vi "BioFeedback13(Small Buckets + Envelope).vi"(7 "Frames Per Second":dbl=30.0, 9 "Start Trial":bool, 11 "End Trial":bool, 12 "Data Directory":path, 13 "File Name":string, 14 "Extension":string="_EMG.txt") -> ()   [LabVIEW 2016]
uses:
  <vilib>/Utility/error.llb/DialogType.ctl
  <vilib>/Waveform/WDTOps.llb/WDT Append Waveforms DBL.vi
  <vilib>/Waveform/WDTFileIO.llb/Export Waveforms To Spreadsheet File (1D).vi
  <vilib>/Utility/file.llb/Write Delimited Spreadsheet (string).vi
panel:
  out "EndProcessTic":u32
  out "StartProcessTic":u32
  out "EndRecordTic":u32
  out "startRecordTic":u32
  out "Start UI":timestamp
  out "UI Elapsed Time":u32
  out "End UI":timestamp
  out "End Process":timestamp
  out "Start Process":timestamp
  out "End Record":timestamp
  out "Start Record":timestamp
  out "Process Elapsed Time":u32
  out "Record Elapsed Time":u32
  out "FilteredTrialData":waveform(dbl)[](graph)
  out "FilteredAndRectified":waveform(dbl)[](graph) caption="Filtered and Rectified"
  out "FilteredTrialData":waveform(dbl)[](array[waveform])
  in  "DisplayChannel":dbl
  out "BigWindowTrialData":dbl[][](array[numeric])
  out "DisplayValueByChannel":dbl[](array[numeric])
  out "RmsBufferSize":dbl
  out "RmsBufferIndices":dbl[](array[numeric])
  in  "Big Window Length (s)":dbl=0.5
  out "RmsBuffers":dbl[][](array[numeric])
  out "SmallWindowTrialData":dbl[][](array[numeric])
  out "CurrentRMSByChannel":dbl[](array[numeric])
  out "FilteredBuffer":dbl[][](array[numeric])
  out "Trial Data Column Headers":string[](array[string])
  in  "TrialDataRowHeaders":string[](array[string])=["Wfm1", "Wfm2", "Wfm3", "Wfm4", "Wfm5", "Wfm6", "Wfm7", "Wfm8"]
  out "GetMaxStartTime":timestamp
  in  "SecondsToAcquireMax":dbl=10.0
  in  "NumberOfMaximumsToTake":dbl=3.0
  in  "CurrentMaxIndex":dbl
  out "SignalsMaxArray":dbl[](array[numeric])
  out "SignalMaxTrialsArray":dbl[][](array[numeric])
  in  "%StdDevIndex":dbl=5.0
  in  "Mean%Index":dbl=4.0
  in  "StdDevIndex":dbl=3.0
  in  "MeanIndex":dbl=2.0
  in  "MaxIndex":dbl=1.0
  in  "MinIndex":dbl
  out "Stability Data":dbl[][](array[numeric])
  out "RawTrialData":waveform(dbl)[](array[waveform])
  in  "UI Ampl Error Path":path=path "C:/Users/Tinggroup/Desktop/VRMuscleActivationVisualizer/VRBiofeedback_v2/assets/BiofeedbackAmplitudeError.txt"
  out "DisplayActivation":dbl
  out "Acquiring Max":bool
  in  "resetMax":bool
  in  "startGetMax":bool
  in  "Amplitude Error":dbl
  in  "UI Data Path":path=path "C:/Users/Tinggroup/Desktop/VRMuscleActivationVisualizer/VRBiofeedback_v2/assets/LeftEMGData.txt"
  in  "EMG Input Device\nProduct Type":string="USB-6009"
  out "DisplayBarActivation":dbl(slide) caption="Left" max=1.0 scale=0.0..100.0
  out "Processed8":dbl[](graph)
  out "Processsed7":dbl[](graph)
  out "Processed6":dbl[](graph)
  out "Processed5":dbl[](graph)
  out "Processed4":dbl[](graph)
  out "Processed3":dbl[](graph)
  out "Processed2":dbl[](graph)
  out "Processed1":dbl[](graph)
  out "Raw Trial Data Wfm":waveform(dbl)[](graph)
  in  "UI Percent Path":path=path "C:/Users/Tinggroup/Desktop/VRMuscleActivationVisualizer/VRBiofeedback_v2/assets/BiofeedbackTargetPercentage.txt"
  in  "Target Percentage":dbl=10.0
  out "Trial In Progress":bool
  in  "Lower Cut-Off":dbl=20.0
  in  "Upper Cut-Off":dbl=300.0
  out "raw data":dynamicdata(graph)
  out "FilteredBufferIndices":dbl[](array[numeric])
  out "FilteredBufferSize":dbl
  out "Samples per frame":dbl
  out "Reset Data Acquisition\nAnd UI Updating":bool=TRUE
  in  "Small Window Length (s)":dbl=0.5
  in  "Sample rate (Hz)":dbl=2000.0
  in  "End Program":bool
  # "Saving Trial Data"
  # "Filter and Process Parameters"
  # "Set Target"
  # "Changes are made instantly and cause moving average to reset to zero"
  # "Scale Max"
  # "Channels used in Display"
  # "Analyze Stability of Displayed Data"
  # "Auto Analyze Stability begins calculating stability\nAs soon as dot enters the target zone and stops \nonce the dot leaves the target zone (Not Yet Implemented)"
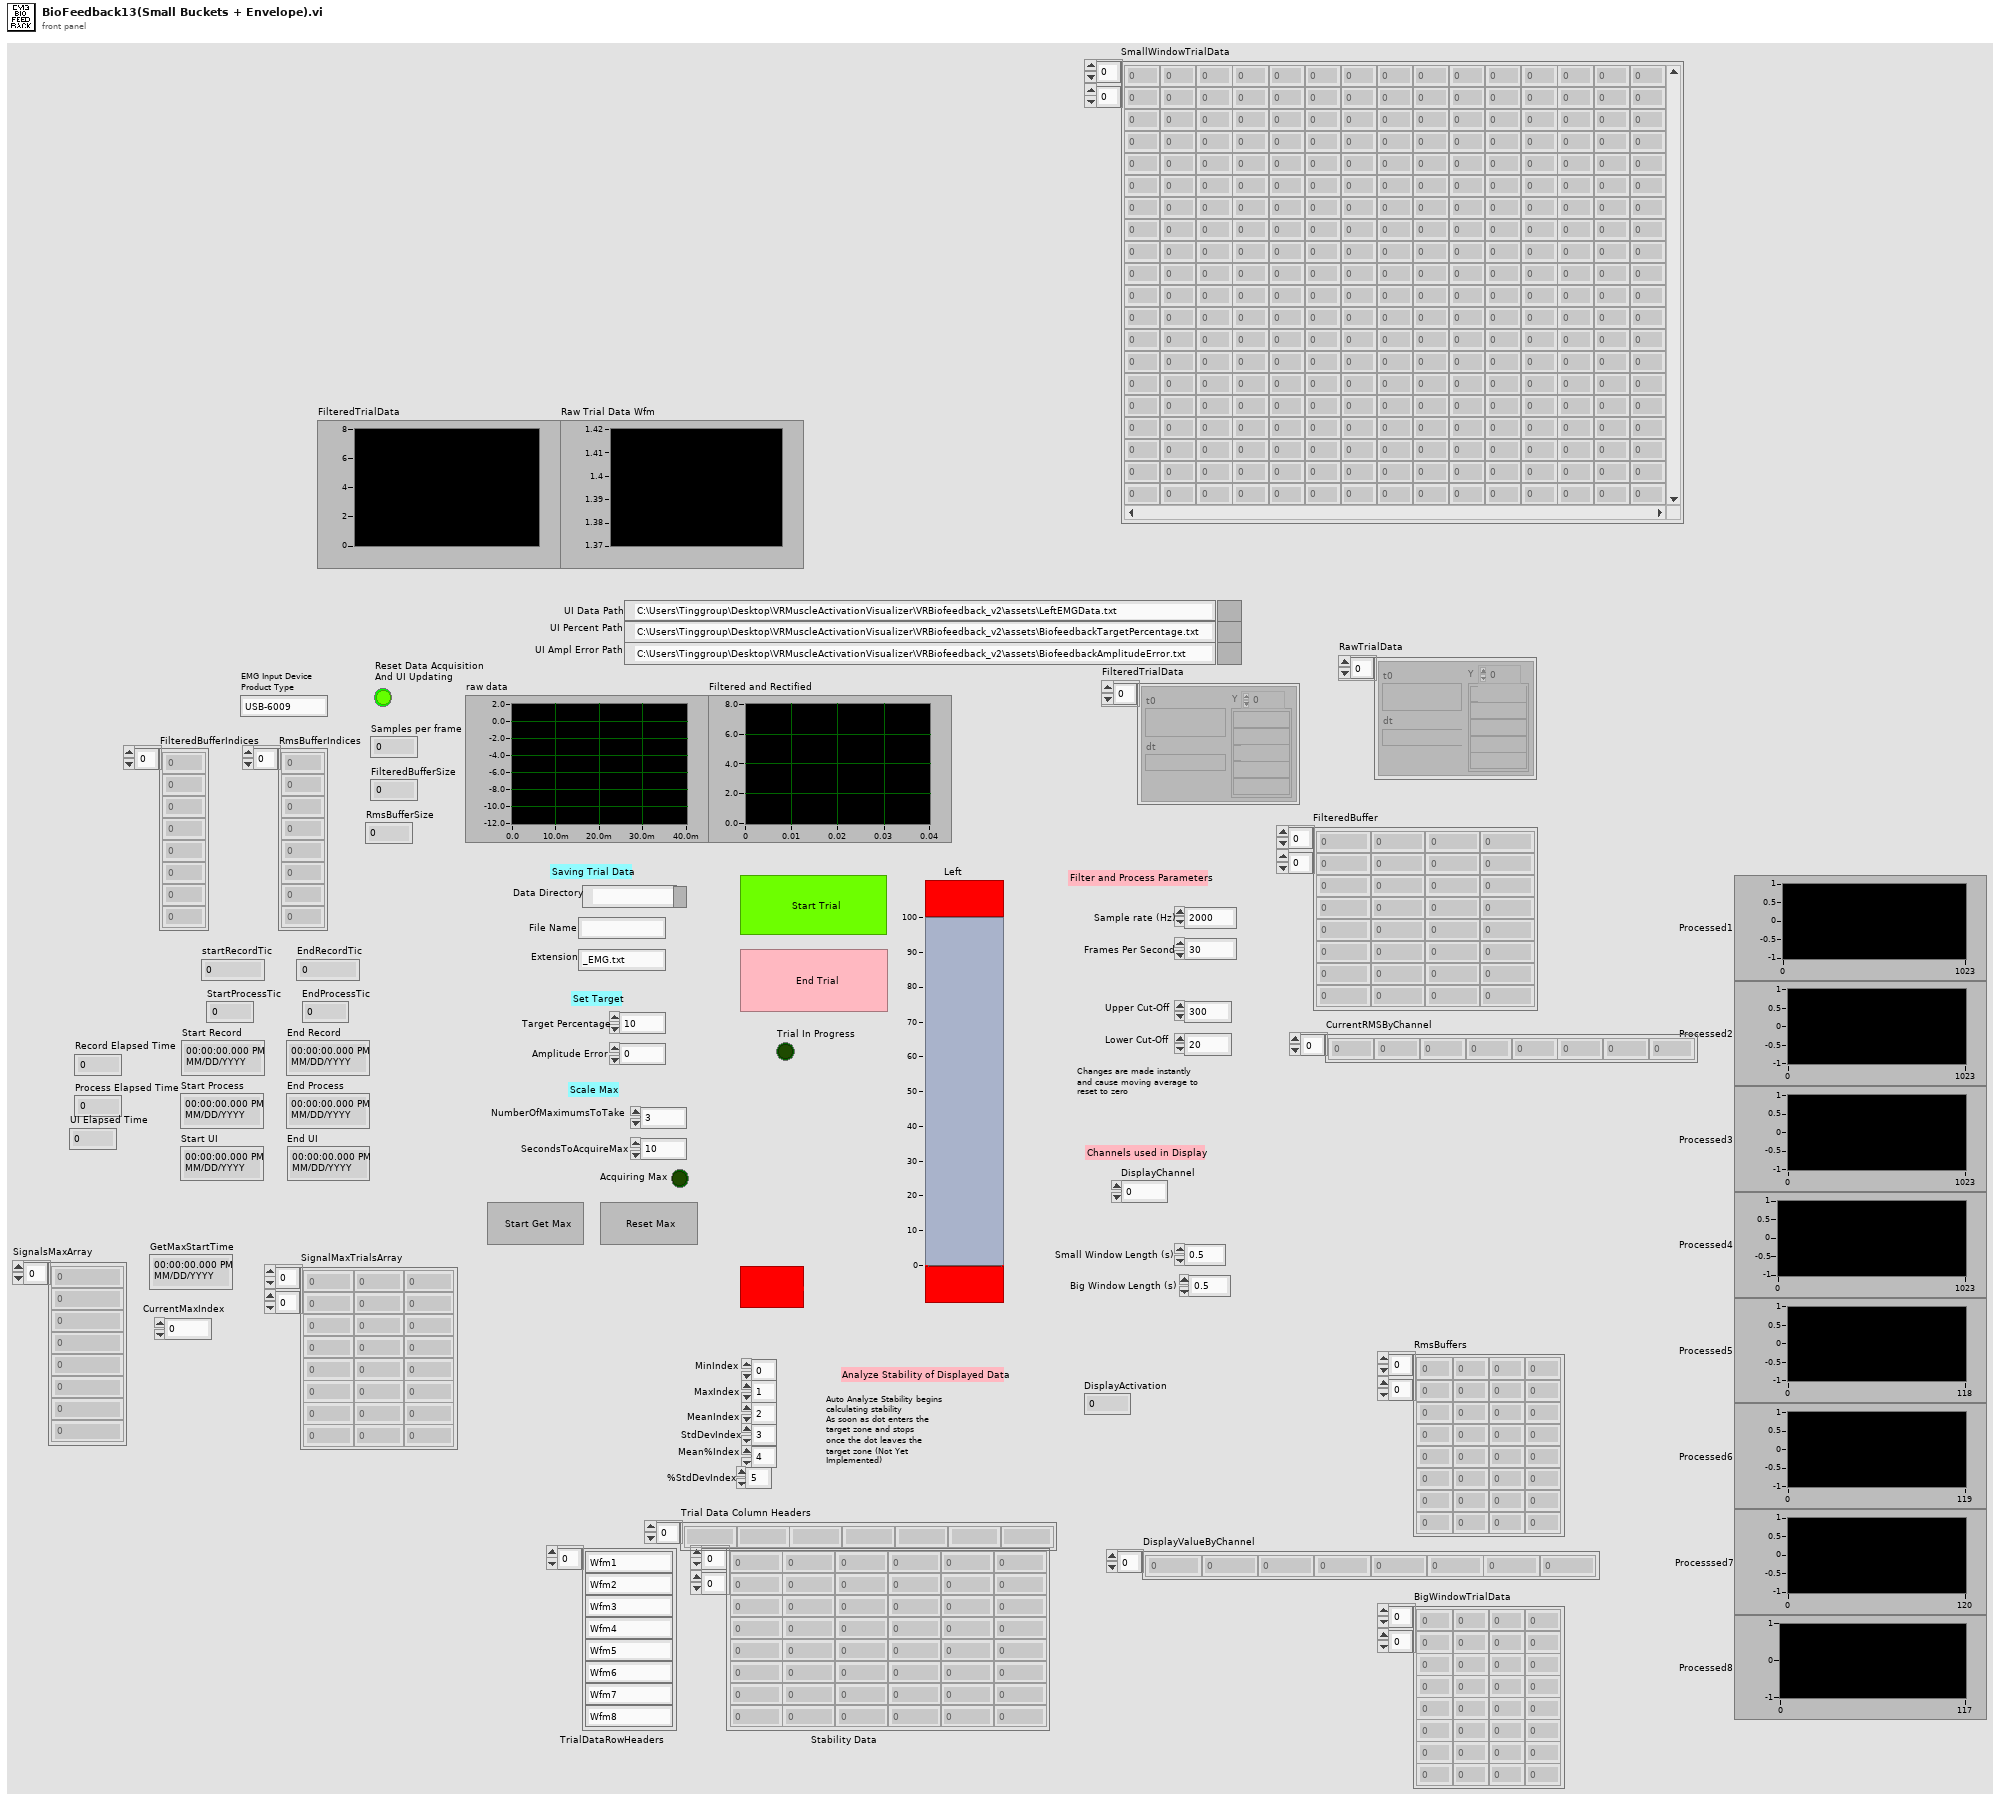
[diagram p1: front panel]
types:
  T1 = typedef "DialogType.ctl" = u16
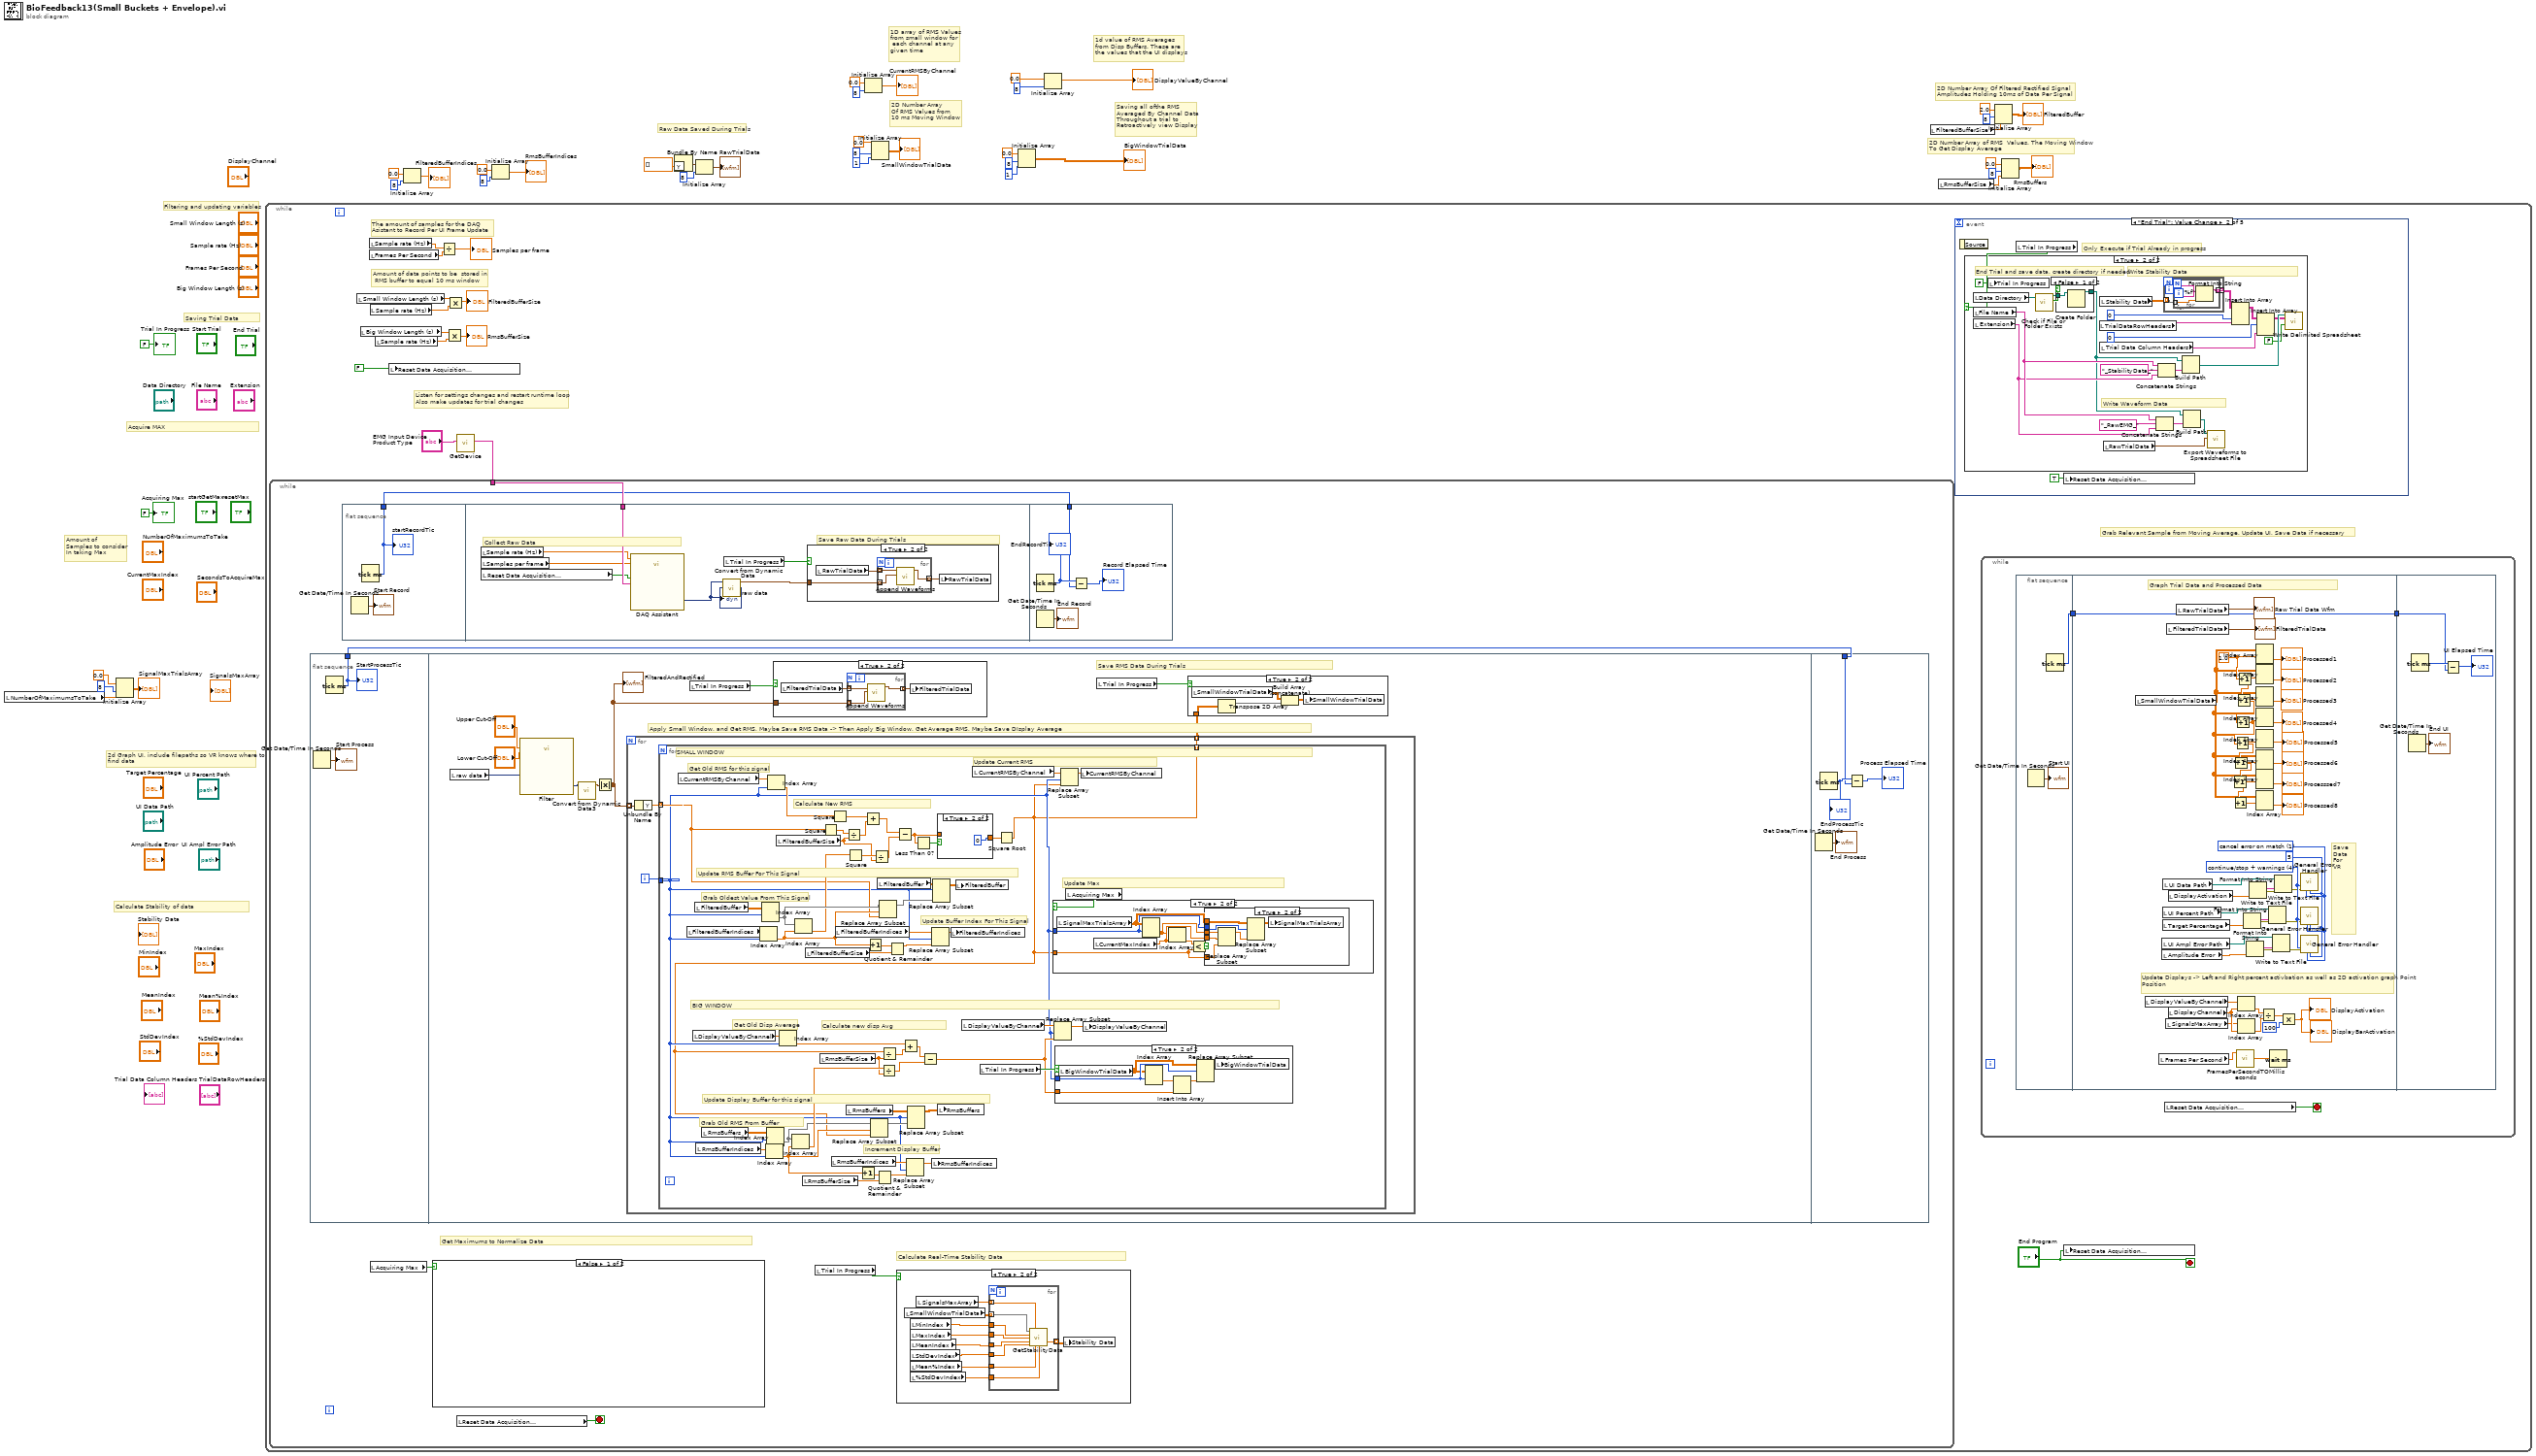
[diagram p0: block diagram]
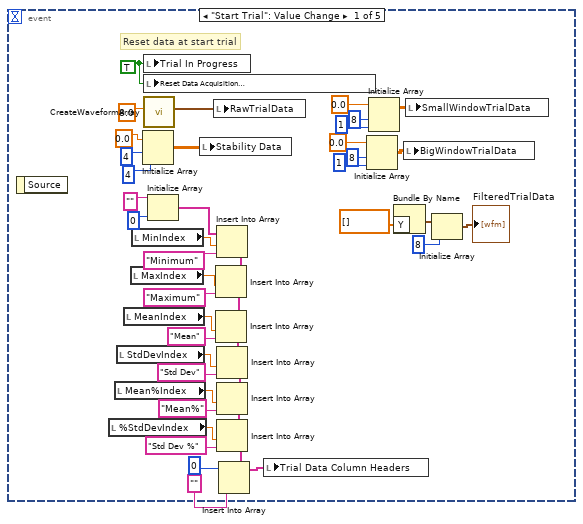
[diagram p2: hidden frame]
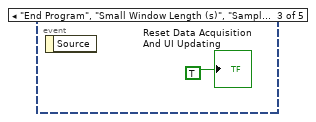
[diagram p5: hidden frame]
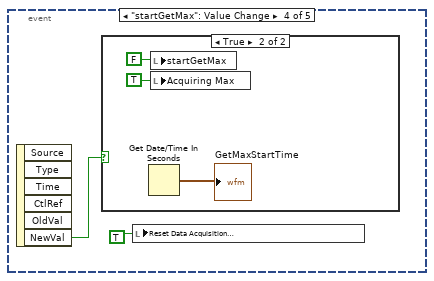
[diagram p6: hidden frame]
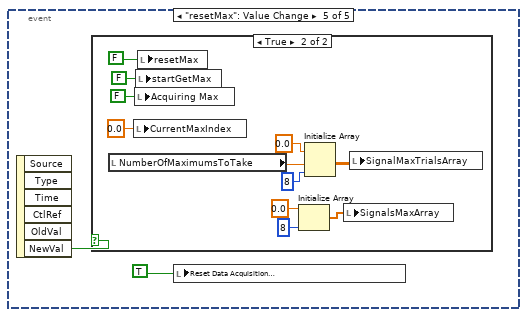
[diagram p8: hidden frame]
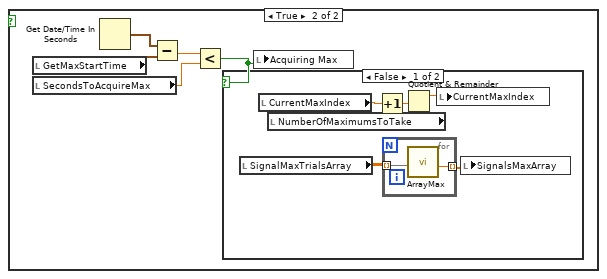
[diagram p17: hidden frame]
diagram:
  # "2D Number Array of RMS  Values. The Moving Window To Get Display Average"
  # "2D Number Array Of Filtered Rectified Signal Amplitudes Holding 10ms of Data Per Signal"
  # "Saving all ofthe RMS\nAveraged By Channel Data\nThroughout a trial to \nRetroactively view Display"
  # "1d value of RMS Averages\nfrom Disp Buffers. These are\nthe values that the UI displays"
  # "1D array of RMS Values\nfrom small window for\n each channel at any\ngiven time"
  # "2D Number Array\nOf RMS Values from\n10 ms Moving Window"
  # "Raw Data Saved During Trials"
  # "Amount of \nSamples to consider\nIn taking Max"
  # "Calculate Stability of data"
  # "Acquire MAX"
  # "Filtering and updating variables"
  # "Saving Trial Data"
  # "2d Graph UI, include filepaths so VR knows where to find data"
  n1 = local read "NumberOfMaximumsToTake"() -> (w12:dbl)
  n2 = Initialize Array(0.0 ("element"), 8 ("dimension size"), w12) -> (→"SignalMaxTrialsArray":dbl[][])
  n3 = while {
    stop <- "End Program" stop-if-true
    # "Grab Relevant Sample from Moving Average, Update UI, Save Data if necessary"
    # "Amount of data points to be  stored in\n RMS buffer to equal 10 ms window"
    # "The amount of samples for the DAQ Asistant to Record Per UI Frame Update"
    # "Listen for settings changes and restart runtime loop\nAlso make updates for trial changes"
    n4 = local read "Small Window Length (s)"() -> (w43:dbl)
    n5 = local read "Big Window Length (s)"() -> (w41:dbl)
    n6 = local read "Sample rate (Hz)"() -> (w51:dbl)
    n7 = local read "Frames Per Second"() -> (w50:dbl)
    n8 = local read "Sample rate (Hz)"() -> (w44:dbl)
    n9 = local read "Sample rate (Hz)"() -> (w40:dbl)
    n10 = local write "Reset Data Acquisition\nAnd UI Updating"(FALSE) -> ()
    n11 = Divide(x=w51, y=w50) -> (x/y=→"Samples per frame":dbl)
    n12 = Multiply(x=w41, y=w40) -> (x*y=→"RmsBufferSize":dbl)
    n13 = Multiply(x=w43, y=w44) -> (x*y=→"FilteredBufferSize":dbl)
    n14 = call "GetDevice.vi"("EMG Input Device\nProduct Type"="EMG Input Device\nProduct Type") -> ("DAQmx Device Name"=w45:tag)  [unwired: 10 in]
    n15 = while {
      tunnel: w45 -> [w209]
      stop <- w204 stop-if-true
      # "Calculate Real-Time Stability Data"
      # "Get Maximums to Normalize Data"
      n16 = flat-sequence {
        tunnel: [w211] -> w206
        tunnel: w206 -> [w312]
        frame #0 {
          n17 = Get Date/Time In Seconds() -> (seconds since 1Jan1904=→"Start Process":timestamp)
          n18 = Tick Count (ms)() -> (millisecond timer value=w211:u32)
          "StartProcessTic" <- w211
        }
        frame #1 {
          # "Save RMS Data During Trials"
          # "Apply Small Window, and Get RMS, Maybe Save RMS Data -> Then Apply Big Window, Get Average RMS, Maybe Save DIsplay Average"
          n19 = local read "raw data"() -> (w220:dynamicdata)
          n20 = call "Filter"("Lower Cut-Off"="Lower Cut-Off", "Upper Cut-Off"="Upper Cut-Off", "Signal"=w220) -> ("Filtered Signal"=w219:dynamicdata)  [unwired: 7 in, 1 out]
          n21 = call "Convert from Dynamic Data3"("Dynamic Data Type"=w219) -> ("Array of Waveform"=w218:waveform(dbl)[])  [unwired: 3 in]
          n22 = Absolute Value(x=w218) -> (abs(x)=w214:waveform(dbl)[])
          "FilteredAndRectified" <- w214
          n23 = for {
            tunnel: w214 -> [w228] mode=indexing
            tunnel: [w225] -> w212 mode=indexing
            i -> [w226]
            n24 = Unbundle By Name(w228) -> ("Y"=w227:dbl[])
            n25 = for {
              tunnel: w227 -> [w238] mode=indexing
              tunnel: w226 -> [w230]
              tunnel: [w229] -> w225 mode=indexing
              # "Update Max"
              # "SMALL WINDOW"
              # "BIG WINDOW"
              # "Increment Display Buffer"
              # "Get Old Disp Average"
              # "Calculate new disp Avg"
              # "Grab Old RMS From Buffer"
              # "Update Display Buffer for this signal"
              # "Update Buffer Index For This Signal"
              # "Update RMS Buffer For This Signal"
              # "Update Current RMS"
              # "Calculate New RMS"
              # "Grab Oldest Value From This Signal"
              # "Get Old RMS for this signal"
              n26 = local read "CurrentRMSByChannel"() -> (w261:dbl[])
              n27 = local read "FilteredBufferIndices"() -> (w266:dbl[])
              n28 = local read "DisplayValueByChannel"() -> (w255:dbl[])
              n29 = local read "FilteredBuffer"() -> (w262:dbl[][])
              n30 = local read "RmsBufferIndices"() -> (w249:dbl[])
              n31 = local read "RmsBuffers"() -> (w258:dbl[][])
              n32 = Index Array(array=w266, index=w230) -> (element=w256:dbl)
              n33 = Index Array(array=w262, index (row)=w230) -> (element=w270:dbl[])  [unwired: 1 in]
              n34 = Index Array(array=w249, index=w230) -> (element=w241:dbl)
              n35 = Index Array(array=w258, index (row)=w230) -> (element=w235:dbl[])  [unwired: 1 in]
              n36 = Index Array(array=w261, index=w230) -> (element=w275:dbl)
              n37 = local read "FilteredBufferSize"() -> (w280:dbl)
              n38 = Index Array(array=w255, index=w230) -> (element=w246:dbl)
              n39 = Index Array(array=w235, index=w241) -> (element=w248:dbl)
              n40 = Index Array(array=w270, index=w256) -> (element=w254:dbl)
              n41 = local read "RmsBufferSize"() -> (w260:dbl)
              n42 = local read "FilteredBufferSize"() -> (w268:dbl)
              n43 = local read "RmsBufferSize"() -> (w245:dbl)
              n44 = Square(x=w238) -> (x^2=w282:dbl)
              n45 = Square(x=w275) -> (x^2=w279:dbl)
              n46 = local read "RmsBufferIndices"() -> (w240:dbl[])
              n47 = local read "FilteredBufferIndices"() -> (w263:dbl[])
              n48 = Divide(x=w282, y=w280) -> (x/y=w278:dbl)
              n49 = local read "RmsBuffers"() -> (w251:dbl[][])
              n50 = Square(x=w254) -> (x^2=w281:dbl)
              n51 = Increment(x=w241) -> (x+1=w259:dbl)
              n52 = Add(x=w279, y=w278) -> (x+y=w277:dbl)
              n53 = Increment(x=w256) -> (x+1=w267:dbl)
              n54 = Divide(x=w281, y=w280) -> (x/y=w276:dbl)
              n55 = Quotient & Remainder(x=w259, y=w260) -> (x-y*floor(x/y)=w239:dbl)  [unwired: 1 out]
              n56 = local read "FilteredBuffer"() -> (w271:dbl[][])
              n57 = Replace Array Subset(array=w270, new element=w238, index=w256) -> (w274:dbl[])
              n58 = Divide(x=w248, y=w245) -> (x/y=w252:dbl)
              n59 = Quotient & Remainder(x=w267, y=w268) -> (x-y*floor(x/y)=w264:dbl)  [unwired: 1 out]
              n60 = Subtract(x=w277, y=w276) -> (x-y=w233:dbl)
              n61 = Replace Array Subset(array=w240, new element=w239, index=w230) -> (w237:dbl[])
              n62 = Less Than 0?(x=w233) -> (x < 0?=w234:bool)
              n63 = Replace Array Subset(array=w263, new element=w264, index=w230) -> (w265:dbl[])
              n64 = local write "RmsBufferIndices"(w237) -> ()
              n65 = Replace Array Subset(array=w271, new element=w274, index (row)=w230) -> (w269:dbl[][])  [unwired: 1 in]
              n66 = case shown="True" w234 {
                tunnel: w233 -> [w297 _]
                tunnel: [w297 0] -> w232
                frame False {
                }
                frame True {
                }
              }
              n67 = local write "FilteredBufferIndices"(w265) -> ()
              n68 = local write "FilteredBuffer"(w269) -> ()
              n69 = local read "DisplayValueByChannel"() -> (w244:dbl[])
              n70 = local read "CurrentRMSByChannel"() -> (w273:dbl[])
              n71 = local read "Trial In Progress"() -> (w242:bool)
              n72 = Square Root(x=w232) -> (sqrt(x)=w229:dbl)
              n73 = Replace Array Subset(array=w235, new element=w229, index=w241) -> (w250:dbl[])
              n74 = Divide(x=w229, y=w245) -> (x/y=w247:dbl)
              n75 = Add(x=w246, y=w247) -> (x+y=w253:dbl)
              n76 = Replace Array Subset(array=w251, new element=w250, index (row)=w230) -> (w257:dbl[][])  [unwired: 1 in]
              n77 = Subtract(x=w253, y=w252) -> (x-y=w236:dbl)
              n78 = local write "RmsBuffers"(w257) -> ()
              n79 = Replace Array Subset(array=w244, new element=w236, index=w230) -> (w243:dbl[])
              n80 = case shown="True" w242 {
                tunnel: w230 -> [_ w302]
                tunnel: w236 -> [_ w303]
                frame False {
                }
                frame True {
                  n81 = local read "BigWindowTrialData"() -> (w301:dbl[][])
                  n82 = Index Array(array=w301, index (row)=w302) -> (element=w304:dbl[])  [unwired: 1 in]
                  n83 = Insert Into Array(array=w304, new element=w303) -> (w300:dbl[])  [unwired: 1 in]
                  n84 = Replace Array Subset(array=w301, new element=w300, index (row)=w302) -> (w299:dbl[][])  [unwired: 1 in]
                  n85 = local write "BigWindowTrialData"(w299) -> ()
                }
              }
              n86 = Replace Array Subset(array=w273, new element=w229, index=w230) -> (w272:dbl[])
              n87 = local read "Acquiring Max"() -> (w231:bool)
              n88 = case shown="True" w231 {
                tunnel: w230 -> [_ w283]
                tunnel: w229 -> [_ w286]
                frame False {
                }
                frame True {
                  n89 = local read "SignalMaxTrialsArray"() -> (w284:dbl[][])
                  n90 = local read "CurrentMaxIndex"() -> (w287:dbl)
                  n91 = Index Array(array=w284, index (row)=w283) -> (element=w285:dbl[])  [unwired: 1 in]
                  n92 = Index Array(array=w285, index=w287) -> (element=w289:dbl)
                  n93 = Less?(x=w289, y=w286) -> (x < y?=w288:bool)
                  n94 = case shown="True" w288 {
                    tunnel: w287 -> [_ w296]
                    tunnel: w286 -> [_ w295]
                    tunnel: w285 -> [_ w294]
                    tunnel: w284 -> [_ w293]
                    tunnel: w283 -> [_ w292]
                    frame False {
                    }
                    frame True {
                      n95 = Replace Array Subset(array=w294, new element=w295, index=w296) -> (w291:dbl[])
                      n96 = Replace Array Subset(array=w293, new element=w291, index (row)=w292) -> (w290:dbl[][])  [unwired: 1 in]
                      n97 = local write "SignalMaxTrialsArray"(w290) -> ()
                    }
                  }
                }
              }
              n98 = local write "CurrentRMSByChannel"(w272) -> ()
              n99 = local write "DisplayValueByChannel"(w243) -> ()
            }
          }
          n100 = local read "Trial In Progress"() -> (w215:bool)
          n101 = case shown="True" w215 {
            tunnel: w214 -> [_ w306]
            frame False {
            }
            frame True {
              n102 = local read "FilteredTrialData"() -> (w307:waveform(dbl)[])
              n103 = for {
                tunnel: w307 -> [w310] mode=indexing
                tunnel: w306 -> [w309] mode=indexing
                tunnel: [w308] -> w305 mode=indexing
                n104 = call-poly <vilib>:"Append Waveforms.vi"("waveform B"=w309, "waveform A"=w310) -> ("waveform out"=w308:waveform(dbl))  [unwired: 8 in, 1 out]
              }
              n105 = local write "FilteredTrialData"(w305) -> ()
            }
          }
          n106 = local read "Trial In Progress"() -> (w213:bool)
          n107 = case shown="True" w213 {
            tunnel: w212 -> [_ w221]
            frame False {
            }
            frame True {
              n108 = local read "SmallWindowTrialData"() -> (w222:dbl[][])
              n109 = Transpose 2D Array(2D array=w221) -> (transposed array=w224:dbl[][])
              n110 = Build Array (concatenate)(w222, w224) -> (w223:dbl[][])
              n111 = local write "SmallWindowTrialData"(w223) -> ()
            }
          }
        }
        frame #2 {
          n112 = Get Date/Time In Seconds() -> (seconds since 1Jan1904=→"End Process":timestamp)
          n113 = Tick Count (ms)() -> (millisecond timer value=w313:u32)
          "EndProcessTic" <- w313
          n114 = Subtract(x=w313, y=w312) -> (x-y=→"Process Elapsed Time":u32)
        }
      }
      n115 = flat-sequence {
        tunnel: [w316] -> w205
        tunnel: w209 -> [w323]
        tunnel: w205 -> [w330]
        frame #0 {
          n116 = Get Date/Time In Seconds() -> (seconds since 1Jan1904=→"Start Record":timestamp)
          n117 = Tick Count (ms)() -> (millisecond timer value=w316:u32)
          "startRecordTic" <- w316
        }
        frame #1 {
          # "Save Raw Data During Trials"
          # "Collect Raw Data"
          n118 = local read "Sample rate (Hz)"() -> (w319:dbl)
          n119 = local read "Samples per frame"() -> (w318:dbl)
          n120 = local read "Reset Data Acquisition\nAnd UI Updating"() -> (w317:bool)
          n121 = call "DAQ Assistant"("rate"=w319, "number of samples"=w318, "stop (T)"=w317, "device name"=w323) -> ("data"=w321:dynamicdata)  [unwired: 13 in, 2 out]
          "raw data" <- w321
          n122 = call "Convert from Dynamic Data"("Dynamic Data Type"=w321) -> ("Array of Waveform"=w320:waveform(dbl)[])  [unwired: 3 in]
          n123 = local read "Trial In Progress"() -> (w322:bool)
          n124 = case shown="True" w322 {
            tunnel: w320 -> [_ w326]
            frame False {
            }
            frame True {
              n125 = local read "RawTrialData"() -> (w325:waveform(dbl)[])
              n126 = for {
                tunnel: w326 -> [w328] mode=indexing
                tunnel: w325 -> [w329] mode=indexing
                tunnel: [w327] -> w324 mode=indexing
                n127 = call-poly <vilib>:"Append Waveforms.vi"("waveform B"=w328, "waveform A"=w329) -> ("waveform out"=w327:waveform(dbl))  [unwired: 8 in, 1 out]
              }
              n128 = local write "RawTrialData"(w324) -> ()
            }
          }
        }
        frame #2 {
          n129 = Get Date/Time In Seconds() -> (seconds since 1Jan1904=→"End Record":timestamp)
          n130 = Tick Count (ms)() -> (millisecond timer value=w331:u32)
          "EndRecordTic" <- w331
          n131 = Subtract(x=w331, y=w330) -> (x-y=→"Record Elapsed Time":u32)
        }
      }
      n132 = local read "Acquiring Max"() -> (w208:bool)
      n133 = case shown="False" w208 {
        frame False {
        }
        frame True {
          n134 = local read "GetMaxStartTime"() -> (w338:timestamp)
          n135 = local read "SecondsToAcquireMax"() -> (w335:dbl)
          n136 = Get Date/Time In Seconds() -> (seconds since 1Jan1904=w337:timestamp)
          n137 = Subtract(x=w337, y=w338) -> (x-y=w336:dbl)
          n138 = Less?(x=w336, y=w335) -> (x < y?=w334:bool)
          n139 = case shown="False" w334 {
            frame False {
              n140 = local read "SignalMaxTrialsArray"() -> (w340:dbl[][])
              n141 = local read "CurrentMaxIndex"() -> (w342:dbl)
              n142 = local read "NumberOfMaximumsToTake"() -> (w344:dbl)
              n143 = Increment(x=w342) -> (x+1=w343:dbl)
              n144 = for {
                tunnel: w340 -> [w346] mode=indexing
                tunnel: [w345] -> w339 mode=indexing
                n145 = call "ArrayMax.vi"("Array"=w346) -> ("max"=w345:dbl)  [unwired: 10 in]
              }
              n146 = Quotient & Remainder(x=w343, y=w344) -> (x-y*floor(x/y)=w341:dbl)  [unwired: 1 out]
              n147 = local write "CurrentMaxIndex"(w341) -> ()
              n148 = local write "SignalsMaxArray"(w339) -> ()
            }
            frame True {
            }
          }
          n149 = local write "Acquiring Max"(w334) -> ()
        }
      }
      n150 = local read "Reset Data Acquisition\nAnd UI Updating"() -> (w204:bool)
      n151 = local read "Trial In Progress"() -> (w207:bool)
      n152 = case shown="True" w207 {
        frame False {
        }
        frame True {
          n153 = local read "SmallWindowTrialData"() -> (w355:dbl[][])
          n154 = local read "MinIndex"() -> (w354:dbl)
          n155 = local read "MaxIndex"() -> (w353:dbl)
          n156 = local read "MeanIndex"() -> (w352:dbl)
          n157 = local read "StdDevIndex"() -> (w351:dbl)
          n158 = local read "Mean%Index"() -> (w350:dbl)
          n159 = local read "%StdDevIndex"() -> (w349:dbl)
          n160 = local read "SignalsMaxArray"() -> (w347:dbl[])
          n161 = for {
            tunnel: w355 -> [w356] mode=indexing
            tunnel: [w357] -> w348 mode=indexing
            tunnel: w354 -> [w364]
            tunnel: w353 -> [w363]
            tunnel: w352 -> [w362]
            tunnel: w351 -> [w361]
            tunnel: w350 -> [w360]
            tunnel: w349 -> [w359]
            tunnel: w347 -> [w358] mode=indexing
            n162 = call "GetStabilityData.vi"("ProvidedData"=w356, "ScaleMax"=w358, "MinIndex"=w364, "MaxIndex"=w363, "MeanIndex"=w362, "StdDevIndex"=w361, "Mean%Index"=w360, "%StdDevIndex"=w359) -> ("ReturnData"=w357:dbl[])  [unwired: 7 in]
          }
          n163 = local write "Stability Data"(w348) -> ()
        }
      }
    }
    n164 = event shown="[1] \"End Trial\": Value Change" {
      selector: _ -> [_ _ _ _ _]
      dyn-events: _ -> [_ _ _ _ _]
      timeout: _ -> [_ _ _ _ _]
      event "Start Trial": Value Change {
        w151 = TRUE ("Trial In Progress")
        # "Reset data at start trial"
        n165 = event-data() -> ()  [unwired: 1 in, 1 out]
        n166 = local read "%StdDevIndex"() -> (w127:dbl)
        n167 = local read "Mean%Index"() -> (w128:dbl)
        n168 = local read "StdDevIndex"() -> (w132:dbl)
        n169 = local read "MeanIndex"() -> (w136:dbl)
        n170 = local read "MaxIndex"() -> (w139:dbl)
        n171 = local read "MinIndex"() -> (w141:dbl)
        n172 = Initialize Array(0.0 ("element"), 4 ("dimension size"), 4 ("dimension size")) -> (w145:dbl[][])
        n173 = local write "Trial In Progress"(w151) -> ()
        n174 = local write "Reset Data Acquisition\nAnd UI Updating"(w151) -> ()
        n175 = call "CreateWaveformArray.vi"("bufferSize"=8.0) -> ("initialized array"=w150:waveform(dbl)[])  [unwired: 5 in, 1 out]
        n176 = Initialize Array("", 0 ("dimension size")) -> (w140:string[])
        n177 = local write "Stability Data"(w145) -> ()
        n178 = local write "RawTrialData"(w150) -> ()
        n179 = Insert Into Array(array=w140, index=w141, new element="Minimum" ("new element/subarray")) -> (w137:string[])
        n180 = Insert Into Array(array=w137, index=w139, new element="Maximum" ("new element/subarray")) -> (w134:string[])
        n181 = Insert Into Array(array=w134, index=w136, new element="Mean" ("new element/subarray")) -> (w131:string[])
        n182 = Insert Into Array(array=w131, index=w132, new element="Std Dev" ("new element/subarray")) -> (w129:string[])
        n183 = Insert Into Array(array=w129, index=w128, new element="Mean%" ("new element/subarray")) -> (w125:string[])
        n184 = Insert Into Array(array=w125, index=w127, new element="Std Dev %" ("new element/subarray")) -> (w122:string[])
        n185 = Insert Into Array(array=w122, index=0, new element="" ("new element/subarray")) -> (w123:string[])
        n186 = local write "Trial Data Column Headers"(w123) -> ()
        n187 = Initialize Array(0.0 ("element"), 8 ("dimension size"), 1 ("dimension size")) -> (w113:dbl[][])
        n188 = Initialize Array(0.0 ("element"), 8 ("dimension size"), 1 ("dimension size")) -> (w120:dbl[][])
        n189 = Bundle By Name("Y"=dbl[] []) -> (w111:waveform(dbl))  [unwired: 1 in]
        n190 = local write "BigWindowTrialData"(w113) -> ()
        n191 = local write "SmallWindowTrialData"(w120) -> ()
        n192 = Initialize Array(w111, 8 ("dimension size")) -> (→"FilteredTrialData":waveform(dbl)[])
      }
      event "End Trial": Value Change {
        # "Only Execute if Trial Already in progress"
        n193 = event-data() -> ()  [unwired: 1 in, 1 out]
        n194 = local read "Trial In Progress"() -> (w153:bool)
        n195 = case shown="True" w153 {
          frame False {
          }
          frame True {
            # "Write Waveform Data"
            # "Write Stability Data"
            # "End Trial and save data, create directory if needed"
            n196 = local read "Data Directory"() -> (w173:path)
            n197 = local read "File Name"() -> (w159:string)
            n198 = local read "Extension"() -> (w158:string)
            n199 = local write "Trial In Progress"(FALSE ("Trial In Progress")) -> ()
            n200 = call <vilib>:"Check if File or Folder Exists.vi"("path"=w173) -> ("file or folder exists?"=w175:bool, "dup path"=w174:path)  [unwired: 8 in, 1 out]
            n201 = case shown="False" w175 {
              tunnel: [w182 w184] -> w157
              tunnel: w174 -> [w183 w184]
              frame False {
                n202 = Create Folder(path (use dialog)=w183) -> (created path=w182:path)  [unwired: 2 in, 2 out]
              }
              frame True {
              }
            }
            n203 = local read "TrialDataRowHeaders"() -> (w168:string[])
            n204 = local read "Stability Data"() -> (w165:dbl[][])
            n205 = local read "Trial Data Column Headers"() -> (w169:string[])
            n206 = local read "RawTrialData"() -> (w155:waveform(dbl)[])
            n207 = Concatenate Strings(w159, "_RawEMG_" ("string"), w158) -> (w156:string)
            n208 = Concatenate Strings(w159, "_StabilityData_" ("string"), w158) -> (w161:string)
            n209 = for {
              tunnel: w165 -> [w178] mode=indexing
              tunnel: [w177] -> w163 mode=indexing
              n210 = for {
                tunnel: w178 -> [w180] mode=indexing
                tunnel: [w179] -> w177 mode=indexing
                n211 = Format Into String(format string="%f", w180) -> (resulting string=w179:string)  [unwired: 2 in, 1 out]
              }
            }
            n212 = Build Path(base path=w157, name or relative path=w161) -> (appended path=w171:path)
            n213 = Build Path(base path=w157, name or relative path=w156) -> (appended path=w154:path)
            n214 = call-poly <vilib>:"Export Waveforms to Spreadsheet File.vi"("waveforms"=w155, "file path (dialog if empty)"=w154) -> ()  [unwired: 8 in, 2 out]
            n215 = Insert Into Array(array=w163, index (col)=0 ("index (row)"), new element=w168) -> (w172:string[][])  [unwired: 1 in]
            n216 = Insert Into Array(array=w172, index (row)=0 ("index (col)"), new element=w169) -> (w164:string[][])  [unwired: 1 in]
            n217 = call-poly <vilib>:"Write Delimited Spreadsheet.vi"("file path (dialog if empty)"=w171, "2D data"=w164, "append to file? (new file:F)"=FALSE) -> ()  [unwired: 11 in, 2 out]
          }
        }
        n218 = local write "Reset Data Acquisition\nAnd UI Updating"(TRUE ("Reset Data Acquisition\nAnd UI Updating")) -> ()
      }
      event "End Program", "Small Window Length (s)", "Sample rate (Hz)", "Frames Per Second": Value Change {
        n219 = event-data() -> ()  [unwired: 1 in, 1 out]
        "Reset Data Acquisition\nAnd UI Updating" <- TRUE
      }
      event "startGetMax": Value Change {
        n220 = event-data() -> ("NewVal"=w187:bool)  [unwired: 1 in, 5 out]
        n221 = case shown="True" w187 {
          frame False {
          }
          frame True {
            n222 = Get Date/Time In Seconds() -> (seconds since 1Jan1904=→"GetMaxStartTime":timestamp)
            n223 = local write "startGetMax"(FALSE) -> ()
            n224 = local write "Acquiring Max"(TRUE ("Acquiring Max")) -> ()
          }
        }
        n225 = local write "Reset Data Acquisition\nAnd UI Updating"(TRUE ("Reset Data Acquisition\nAnd UI Updating")) -> ()
      }
      event "resetMax": Value Change {
        n226 = event-data() -> ("NewVal"=w192:bool)  [unwired: 1 in, 5 out]
        n227 = case shown="True" w192 {
          frame False {
          }
          frame True {
            n228 = local read "NumberOfMaximumsToTake"() -> (w198:dbl)
            n229 = local write "CurrentMaxIndex"(0.0 ("CurrentMaxIndex")) -> ()
            n230 = local write "Acquiring Max"(FALSE ("Acquiring Max")) -> ()
            n231 = local write "startGetMax"(FALSE ("startGetMax")) -> ()
            n232 = local write "resetMax"(FALSE ("endGetMax")) -> ()
            n233 = Initialize Array(0.0 ("element"), 8 ("dimension size")) -> (w194:dbl[])
            n234 = Initialize Array(0.0 ("element"), w198, 8 ("dimension size")) -> (w199:dbl[][])
            n235 = local write "SignalsMaxArray"(w194) -> ()
            n236 = local write "SignalMaxTrialsArray"(w199) -> ()
          }
        }
        n237 = local write "Reset Data Acquisition\nAnd UI Updating"(TRUE ("Reset Data Acquisition\nAnd UI Updating")) -> ()
      }
    }
    n238 = while {
      stop <- w52 stop-if-true
      n239 = flat-sequence {
        tunnel: [w56] -> w54
        tunnel: [w104] -> w53
        tunnel: w54 -> [w104]
        tunnel: w53 -> [w105]
        frame #0 {
          n240 = Get Date/Time In Seconds() -> (seconds since 1Jan1904=→"Start UI":timestamp)
          n241 = Tick Count (ms)() -> (millisecond timer value=w56:u32)
        }
        frame #1 {
          w97 = 1.0 ("x")
          w77 = T1 4 items=["no dialog", "OK message", "continue or stop message", "OK message + warnings", "continue/stop + warnings"] ("type of dialog (OK msg:1)")
          w78 = 1 items=["no exception", "cancel error on match", "set error on match"] ("[exception action] (none:0)")
          w79 = 5 ("[exception code]")
          # "Graph Trial Data and Processed Data"
          # "Update Displays -> Left and Right percent activbation as well as 2D activation graph Point Position"
          # "Save\nData\nFor\nVR"
          n242 = local read "SmallWindowTrialData"() -> (w88:dbl[][])
          n243 = local read "DisplayValueByChannel"() -> (w98:dbl[])
          n244 = local read "Frames Per Second"() -> (w57:dbl)
          n245 = local read "UI Ampl Error Path"() -> (w76:path)
          n246 = local read "Amplitude Error"() -> (w75:dbl)
          n247 = local read "UI Percent Path"() -> (w67:path)
          n248 = local read "Target Percentage"() -> (w68:dbl)
          n249 = local read "UI Data Path"() -> (w60:path)
          n250 = local read "SignalsMaxArray"() -> (w99:dbl[])
          n251 = local read "FilteredTrialData"() -> (→"FilteredTrialData":waveform(dbl)[])
          n252 = local read "DisplayActivation"() -> (w62:dbl)
          n253 = local read "DisplayChannel"() -> (w100:dbl)
          n254 = local read "RawTrialData"() -> (→"Raw Trial Data Wfm":waveform(dbl)[])
          n255 = Increment(x=w97) -> (x+1=w96:dbl)
          n256 = Increment(x=w96) -> (x+1=w95:dbl)
          n257 = Increment(x=w95) -> (x+1=w94:dbl)
          n258 = Increment(x=w94) -> (x+1=w93:dbl)
          n259 = Increment(x=w93) -> (x+1=w92:dbl)
          n260 = Increment(x=w92) -> (x+1=w91:dbl)
          n261 = Increment(x=w91) -> (x+1=w90:dbl)
          n262 = call "FramesPerSecondTOMilliseconds.vi"("Thermometer\nFps"=w57) -> ("x*y"=w80:dbl)  [unwired: 10 in]
          n263 = Index Array(array=w98, index=w100) -> (element=w101:dbl)
          n264 = Index Array(array=w99, index=w100) -> (element=w102:dbl)
          n265 = Format Into String(w68) -> (resulting string=w66:string, error out=w65:errorcluster)  [unwired: 3 in]
          n266 = Format Into String(w75) -> (resulting string=w74:string, error out=w73:errorcluster)  [unwired: 3 in]
          n267 = Format Into String(w62) -> (resulting string=w61:string, error out=w59:errorcluster)  [unwired: 3 in]
          n268 = Index Array(array=w88, index (row)=w97) -> (element=→"Processed1":dbl[])  [unwired: 1 in]
          n269 = Index Array(array=w88, index (row)=w96) -> (element=→"Processed2":dbl[])  [unwired: 1 in]
          n270 = Index Array(array=w88, index (row)=w95) -> (element=→"Processed3":dbl[])  [unwired: 1 in]
          n271 = Index Array(array=w88, index (row)=w94) -> (element=→"Processed4":dbl[])  [unwired: 1 in]
          n272 = Index Array(array=w88, index (row)=w93) -> (element=→"Processed5":dbl[])  [unwired: 1 in]
          n273 = Index Array(array=w88, index (row)=w92) -> (element=→"Processed6":dbl[])  [unwired: 1 in]
          n274 = Index Array(array=w88, index (row)=w91) -> (element=→"Processsed7":dbl[])  [unwired: 1 in]
          n275 = Index Array(array=w88, index (row)=w90) -> (element=→"Processed8":dbl[])  [unwired: 1 in]
          n276 = Divide(x=w101, y=w102) -> (x/y=w70:dbl)
          n277 = Write to Text File(file (use dialog)=w67, text=w66, error in=w65) -> (error out=w64:errorcluster)  [unwired: 1 in, 2 out]
          n278 = Wait (ms)(milliseconds to wait=w80) -> ()  [unwired: 1 out]
          n279 = Write to Text File(file (use dialog)=w76, text=w74, error in=w73) -> (error out=w72:errorcluster)  [unwired: 1 in, 2 out]
          n280 = Write to Text File(file (use dialog)=w60, text=w61, error in=w59) -> (error out=w58:errorcluster)  [unwired: 1 in, 2 out]
          n281 = Multiply(x=w70, y=100) -> (x*y=→"DisplayBarActivation" →"DisplayActivation":dbl)
          n282 = call <vilib>:"General Error Handler.vi"("type of dialog (OK msg:1)"=w77, "error in (no error)"=w58, "[exception action] (none:0)"=w78, "[exception code]"=w79) -> ()  [unwired: 7 in, 5 out]
          n283 = call <vilib>:"General Error Handler.vi"("type of dialog (OK msg:1)"=w77, "error in (no error)"=w64, "[exception action] (none:0)"=w78, "[exception code]"=w79) -> ()  [unwired: 7 in, 5 out]
          n284 = call <vilib>:"General Error Handler.vi"("type of dialog (OK msg:1)"=w77, "error in (no error)"=w72, "[exception action] (none:0)"=w78, "[exception code]"=w79) -> ()  [unwired: 7 in, 5 out]
        }
        frame #2 {
          n285 = Get Date/Time In Seconds() -> (seconds since 1Jan1904=→"End UI":timestamp)
          n286 = Tick Count (ms)() -> (millisecond timer value=w106:u32)
          n287 = Subtract(x=w106, y=w105) -> (x-y=→"UI Elapsed Time":u32)
        }
      }
      n288 = local read "Reset Data Acquisition\nAnd UI Updating"() -> (w52:bool)
    }
    n289 = local write "Reset Data Acquisition\nAnd UI Updating"("End Program") -> ()
  }
  n290 = Initialize Array(0.0 ("element"), 8 ("dimension size")) -> (→"FilteredBufferIndices":dbl[])
  n291 = Initialize Array(0.0 ("element"), 8 ("dimension size")) -> (→"RmsBufferIndices":dbl[])
  n292 = Bundle By Name("Y"=dbl[] []) -> (w17:waveform(dbl))  [unwired: 1 in]
  n293 = Initialize Array(w17, 8 ("dimension size")) -> (→"RawTrialData":waveform(dbl)[])
  n294 = Initialize Array(0.0 ("element"), 8 ("dimension size")) -> (→"CurrentRMSByChannel":dbl[])
  n295 = Initialize Array(0.0 ("element"), 8 ("dimension size"), 1 ("dimension size")) -> (→"SmallWindowTrialData":dbl[][])
  n296 = Initialize Array(0.0 ("element"), 8 ("dimension size"), 1 ("dimension size")) -> (→"BigWindowTrialData":dbl[][])
  n297 = Initialize Array(0.0 ("element"), 8 ("dimension size")) -> (→"DisplayValueByChannel":dbl[])
  n298 = local read "FilteredBufferSize"() -> (w11:dbl)
  n299 = local read "RmsBufferSize"() -> (w10:dbl)
  n300 = Initialize Array(2.0 ("element"), 8 ("dimension size"), w11) -> (→"FilteredBuffer":dbl[][])
  n301 = Initialize Array(0.0 ("element"), 8 ("dimension size"), w10) -> (→"RmsBuffers":dbl[][])
  "Trial In Progress" <- FALSE ("Trial In Progress")
  "Acquiring Max" <- FALSE ("Acquiring Max")
